vi "Bounce Path.vi"   [LabVIEW 2019]
uses:
  Robot Global Data.vi
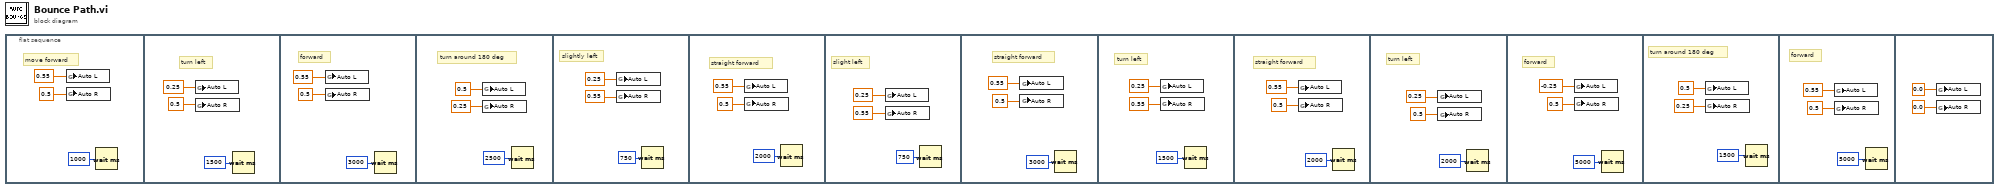
[diagram p0: block diagram]
diagram:
  n1 = flat-sequence {
    frame #0 {
      # "move forward"
      n2 = global write "Robot Global Data.vi" "Auto L"(0.55 ("Joystick X")) -> ()
      n3 = global write "Robot Global Data.vi" "Auto R"(0.5 ("Joystick Y")) -> ()
      n4 = Wait (ms)(milliseconds to wait=u32 1000) -> ()  [unwired: 1 out]
    }
    frame #1 {
      # "turn left"
      n5 = global write "Robot Global Data.vi" "Auto L"(0.25 ("Joystick X")) -> ()
      n6 = global write "Robot Global Data.vi" "Auto R"(0.5 ("Joystick Y")) -> ()
      n7 = Wait (ms)(milliseconds to wait=u32 1500) -> ()  [unwired: 1 out]
    }
    frame #2 {
      # "forward"
      n8 = global write "Robot Global Data.vi" "Auto L"(0.55 ("Joystick X")) -> ()
      n9 = global write "Robot Global Data.vi" "Auto R"(0.5 ("Joystick Y")) -> ()
      n10 = Wait (ms)(milliseconds to wait=u32 3000) -> ()  [unwired: 1 out]
    }
    frame #3 {
      # "turn around 180 deg"
      n11 = global write "Robot Global Data.vi" "Auto L"(0.5 ("Joystick X")) -> ()
      n12 = global write "Robot Global Data.vi" "Auto R"(0.25 ("Joystick Y")) -> ()
      n13 = Wait (ms)(milliseconds to wait=u32 2500) -> ()  [unwired: 1 out]
    }
    frame #4 {
      # "slightly left"
      n14 = global write "Robot Global Data.vi" "Auto L"(0.25 ("Joystick X")) -> ()
      n15 = global write "Robot Global Data.vi" "Auto R"(0.55 ("Joystick Y")) -> ()
      n16 = Wait (ms)(milliseconds to wait=u32 750) -> ()  [unwired: 1 out]
    }
    frame #5 {
      # "straight forward"
      n17 = global write "Robot Global Data.vi" "Auto L"(0.55 ("Joystick X")) -> ()
      n18 = global write "Robot Global Data.vi" "Auto R"(0.5 ("Joystick Y")) -> ()
      n19 = Wait (ms)(milliseconds to wait=u32 2000) -> ()  [unwired: 1 out]
    }
    frame #6 {
      # "slight left"
      n20 = global write "Robot Global Data.vi" "Auto L"(0.25 ("Joystick X")) -> ()
      n21 = global write "Robot Global Data.vi" "Auto R"(0.55 ("Joystick Y")) -> ()
      n22 = Wait (ms)(milliseconds to wait=u32 750) -> ()  [unwired: 1 out]
    }
    frame #7 {
      # "straight forward"
      n23 = global write "Robot Global Data.vi" "Auto L"(0.55 ("Joystick X")) -> ()
      n24 = global write "Robot Global Data.vi" "Auto R"(0.5 ("Joystick Y")) -> ()
      n25 = Wait (ms)(milliseconds to wait=u32 3000) -> ()  [unwired: 1 out]
    }
    frame #8 {
      # "turn left"
      n26 = global write "Robot Global Data.vi" "Auto L"(0.25 ("Joystick X")) -> ()
      n27 = global write "Robot Global Data.vi" "Auto R"(0.55 ("Joystick Y")) -> ()
      n28 = Wait (ms)(milliseconds to wait=u32 1500) -> ()  [unwired: 1 out]
    }
    frame #9 {
      # "straight forward"
      n29 = global write "Robot Global Data.vi" "Auto L"(0.55 ("Joystick X")) -> ()
      n30 = global write "Robot Global Data.vi" "Auto R"(0.5 ("Joystick Y")) -> ()
      n31 = Wait (ms)(milliseconds to wait=u32 2000) -> ()  [unwired: 1 out]
    }
    frame #10 {
      # "turn left"
      n32 = global write "Robot Global Data.vi" "Auto L"(0.25 ("Joystick X")) -> ()
      n33 = global write "Robot Global Data.vi" "Auto R"(0.5 ("Joystick Y")) -> ()
      n34 = Wait (ms)(milliseconds to wait=u32 2000) -> ()  [unwired: 1 out]
    }
    frame #11 {
      # "forward"
      n35 = global write "Robot Global Data.vi" "Auto L"(-0.25 ("Joystick X")) -> ()
      n36 = global write "Robot Global Data.vi" "Auto R"(0.5 ("Joystick Y")) -> ()
      n37 = Wait (ms)(milliseconds to wait=u32 5000) -> ()  [unwired: 1 out]
    }
    frame #12 {
      # "turn around 180 deg"
      n38 = global write "Robot Global Data.vi" "Auto L"(0.5 ("Joystick X")) -> ()
      n39 = global write "Robot Global Data.vi" "Auto R"(0.25 ("Joystick Y")) -> ()
      n40 = Wait (ms)(milliseconds to wait=u32 1500) -> ()  [unwired: 1 out]
    }
    frame #13 {
      # "forward"
      n41 = global write "Robot Global Data.vi" "Auto L"(0.55 ("Joystick X")) -> ()
      n42 = global write "Robot Global Data.vi" "Auto R"(0.5 ("Joystick Y")) -> ()
      n43 = Wait (ms)(milliseconds to wait=u32 5000) -> ()  [unwired: 1 out]
    }
    frame #14 {
      n44 = global write "Robot Global Data.vi" "Auto L"(0.0 ("Joystick X")) -> ()
      n45 = global write "Robot Global Data.vi" "Auto R"(0.0 ("Joystick Y")) -> ()
    }
  }
